vi "MakeArrayRightSize.vi"(6 "Row or Column":enum16{"Rows", "Columns"}(ring), 7 "Max Visible Size":u16, 8 "Size":i16, 9 "Master Array In":variant[](array[variant]), 10 "Array":variant[](array[variant]), 11 "reference":refnum<vi>) -> (2 "Array Out":variant[](array[variant]), 3 "Master Array Out":variant[](array[variant]))   [LabVIEW 2016]
panel:
  out "new array size":i32
  out "master array size":i32
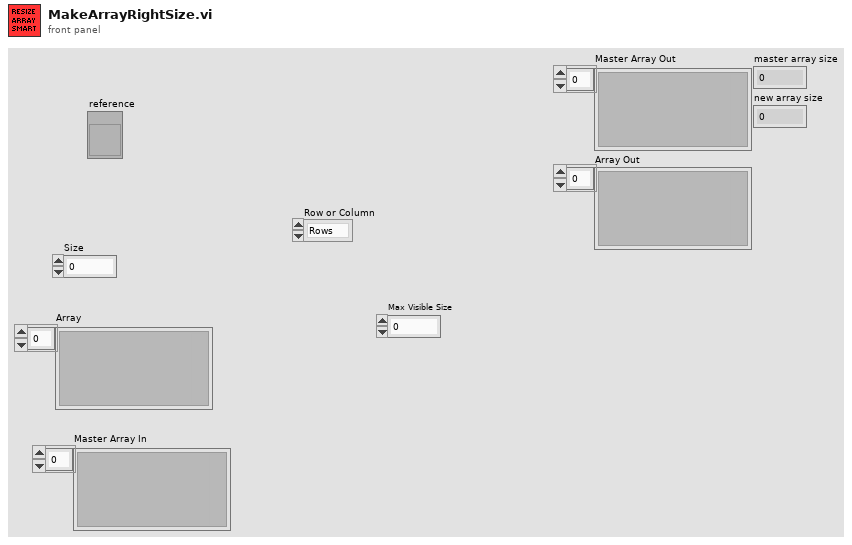
[diagram p1: front panel]
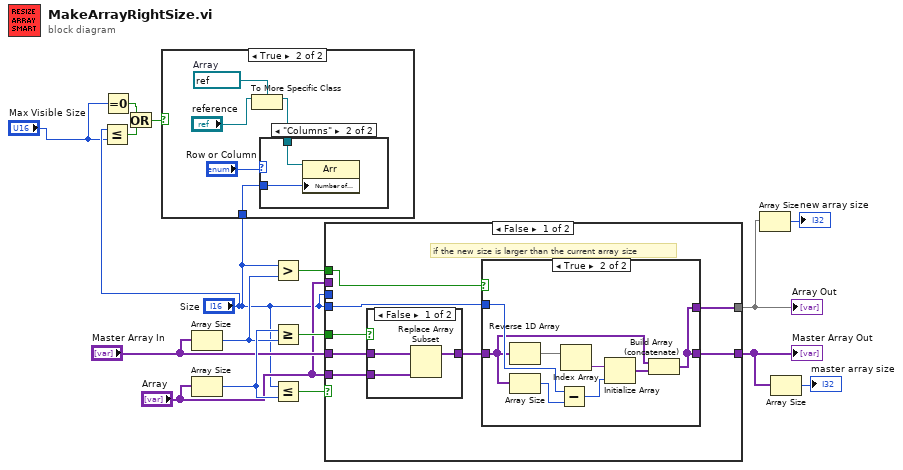
[diagram p0: block diagram]
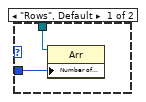
[diagram p3: hidden frame]
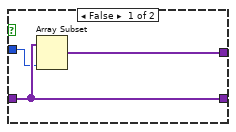
[diagram p5: hidden frame]
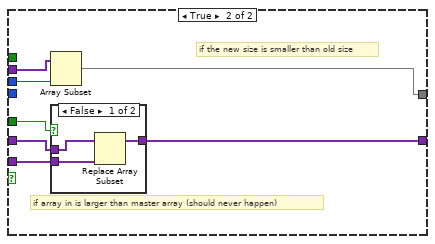
[diagram p6: hidden frame]
diagram:
  n1 = Less Or Equal?(x="Size", y="Max Visible Size") -> (x <= y?=w2:bool)
  n2 = Equal To 0?(x="Max Visible Size") -> (x = 0?=w1:bool)
  n3 = Or(x=w1, y=w2) -> (x .or. y?=w3:bool)
  n4 = case shown="True" w3 {
    tunnel: "Size" -> [_ w21]
    frame False {
    }
    frame True {
      w20 = refnum<vi> refnum  # Array
      n5 = To More Specific Class(target class=w20, reference="reference") -> (specific class reference=w19:refnum<vi>)  [unwired: 1 in, 1 out]
      n6 = case shown="\"Columns\"" "Row or Column" {
        tunnel: w21 -> [w23 w25]
        tunnel: w19 -> [w22 w24]
        frame "Rows", Default {
          n7 = property class="Arr"(reference=w22, "Number of Rows"=w23) -> ()  [unwired: 1 in, 2 out]
        }
        frame "Columns" {
          n8 = property class="Arr"(reference=w24, "Number of Columns"=w25) -> ()  [unwired: 1 in, 2 out]
        }
      }
    }
  }
  n9 = Array Size(array="Master Array In") -> (size(s)=w11:i32)
  n10 = Array Size(array="Array") -> (size(s)=w16:i32)
  n11 = Greater?(x="Size", y=w11) -> (0:w10:bool)
  n12 = Greater Or Equal?(x=w16, y=w11) -> (x >= y?=w14:bool)
  n13 = Less Or Equal?(x="Size", y=w16) -> (x <= y?=w15:bool)
  n14 = case shown="False" w15 {
    tunnel: "Size" -> [_ w55]
    tunnel: "Array" -> [_ w54]
    tunnel: [w27 w53] -> w7
    tunnel: w14 -> [w31 w52]
    tunnel: "Master Array In" -> [w33 w51]
    tunnel: "Array" -> [w32 w50]
    tunnel: [w26 w49] -> w9
    tunnel: w10 -> [w30 _]
    tunnel: "Size" -> [w28 _]
    frame False {
      # "if the new size is larger than the current array size"
      n15 = case shown="False" w31 {
        tunnel: w33 -> [w36 _]
        tunnel: w32 -> [w35 w37]
        tunnel: [w34 w37] -> w29
        frame False {
          n16 = Replace Array Subset(array=w36, new element=w35) -> (w34:variant[])  [unwired: 1 in]
        }
        frame True {
        }
      }
      n17 = case shown="True" w30 {
        tunnel: w29 -> [w40 w42]
        tunnel: w28 -> [w39 w46]
        tunnel: [w38 w41] -> w27
        tunnel: [w40 w41] -> w26
        frame False {
          n18 = Array Subset(array=w40, length=w39) -> (w38:variant[])  [unwired: 1 in]
        }
        frame True {
          n19 = Reverse 1D Array(array=w42) -> (reversed array=w48:variant[])
          n20 = Array Size(array=w42) -> (size(s)=w45:i32)
          n21 = Subtract(x=w46, y=w45) -> (x-y=w44:i32)
          n22 = Index Array(array=w48) -> (element=w47:variant)  [unwired: 1 in]
          n23 = Initialize Array(w47, w44) -> (w43:variant[])
          n24 = Build Array (concatenate)(w42, w43) -> (w41:variant[])
        }
      }
    }
    frame True {
      # "if array in is larger than master array (should never happen)"
      # "if the new size is smaller than old size"
      n25 = Array Subset(array=w54, length=w55) -> (w53:variant[])  [unwired: 1 in]
      n26 = case shown="False" w52 {
        tunnel: w51 -> [w58 _]
        tunnel: w50 -> [w57 w59]
        tunnel: [w56 w59] -> w49
        frame False {
          n27 = Replace Array Subset(array=w58, new element=w57) -> (w56:variant[])  [unwired: 1 in]
        }
        frame True {
        }
      }
    }
  }
  "Master Array Out" <- w9
  "Array Out" <- w7
  n28 = Array Size(array=w7) -> (size(s)=→"new array size":i32)
  n29 = Array Size(array=w9) -> (size(s)=→"master array size":i32)
